vi "Global_Cube_calculationVar.vi"() -> ()   [LabVIEW 2017]
panel:
  in  "Scale factor":dbl
  in  "Deadband":dbl
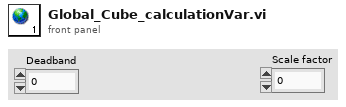
[diagram p1: front panel]
diagram:
